vi "DT3120_ChopU32FromBArray.vi"(11 "BArray In":u8[](array[numeric])) -> (1 "Value":u32, 3 "BArray Out":u8[](array[numeric]))   [LabVIEW 2010]
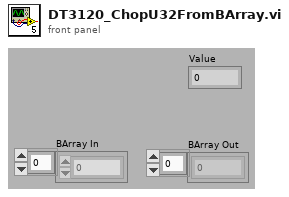
[diagram p1: front panel]
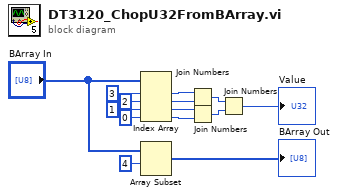
[diagram p0: block diagram]
diagram:
  n1 = Index Array(array="BArray In", index #1=3 ("index"), index #2=2 ("index"), index #3=1 ("index"), index #4=0 ("index")) -> (element #1=w8:u8, element #2=w9:u8, element #3=w10:u8, element #4=w11:u8)
  n2 = Array Subset(array="BArray In", index=4) -> (→"BArray Out":u8[])  [unwired: 1 in]
  n3 = Join Numbers(hi=w8, lo=w9) -> ((hi.lo)=w12:u16)
  n4 = Join Numbers(hi=w10, lo=w11) -> ((hi.lo)=w13:u16)
  n5 = Join Numbers(hi=w12, lo=w13) -> ((hi.lo)=→"Value":u32)
